vi "Initialize.vi"(7 "timeout, ms (2000)":u32=2000, 8 "error in (no error)":errorcluster, 9 "configuration file path":path, 10 "port":refnum<visa-resource-name>, 11 "SOL MS in":refnum<class "PL SOL Instruments MS.lvclass">) -> (0 "error out":errorcluster, 3 "SOL MS out":refnum<class "PL SOL Instruments MS.lvclass">)   [LabVIEW 2015, in "PL SOL Instruments MS.lvclass"]
doc: "Initializes connection to device using specified settings. <b>Configuration file path</b> is a path to the manufacturer .cfg file (e.g. MS3504.cfg) that contains device specification."
uses:
  PL SOL Instruments MS.lvclass
  PL SOL Instruments MS.lvclass/PL SOL Instruments MS.ctl
  <vilib>/Utility/config.llb/Read Key (U32).vi
  <vilib>/Utility/config.llb/Read Key (String).vi
  <vilib>/Utility/config.llb/Read Key (I32).vi
  <vilib>/Utility/config.llb/NI_LVConfig.lvlib
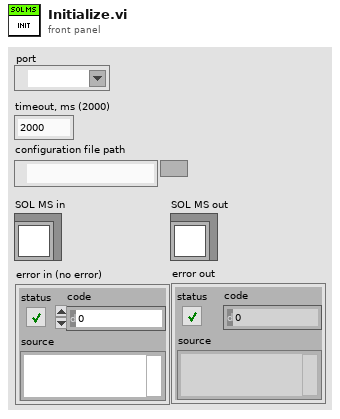
[diagram p1: front panel]
types:
  T1 = typedef "NI_LVConfig.lvlib/Config Data RefNum.ctl" = refnum<k1>
  T2 = cluster{"name":string, "step timeout, ms":u32, "reset timeout, ms":u32, "gratings":cluster{"name":string, "step timeout, ms":u32, "reset timeout, ms":u32, "turret position":i32, "reset position":i32, "max position":i32, "backlash distance":i32, "step size, rad":dbl, "groove density, g/mm":dbl, "theta2, rad":dbl, "blaze wavelength, nm":dbl, "focal length, cm":dbl, "manual change":bool, "manual change position":i32}[], "current grating":cluster{"index":u8, "position":i32}}[]
  T3 = cluster{"name":string, "step timeout, ms":u32, "reset timeout, ms":u32, "gratings":cluster{"name":string, "step timeout, ms":u32, "reset timeout, ms":u32, "turret position":i32, "reset position":i32, "max position":i32, "backlash distance":i32, "step size, rad":dbl, "groove density, g/mm":dbl, "theta2, rad":dbl, "blaze wavelength, nm":dbl, "focal length, cm":dbl, "manual change":bool, "manual change position":i32}[], "current grating":cluster{"index":u8, "position":i32}}
  T4 = cluster{"name":string, "step timeout, ms":u32, "reset timeout, ms":u32, "turret position":i32, "reset position":i32, "max position":i32, "backlash distance":i32, "step size, rad":dbl, "groove density, g/mm":dbl, "theta2, rad":dbl, "blaze wavelength, nm":dbl, "focal length, cm":dbl, "manual change":bool, "manual change position":i32}[]
  T5 = cluster{"name":string, "step timeout, ms":u32, "reset timeout, ms":u32, "turret position":i32, "reset position":i32, "max position":i32, "backlash distance":i32, "step size, rad":dbl, "groove density, g/mm":dbl, "theta2, rad":dbl, "blaze wavelength, nm":dbl, "focal length, cm":dbl, "manual change":bool, "manual change position":i32}
  T6 = cluster{"name":string, "step timeout, ms":u32, "reset timeout, ms":u32, "positions":cluster{"name":string, "position":i32}[], "current position index":u8}[]
  T7 = cluster{"name":string, "step timeout, ms":u32, "reset timeout, ms":u32, "positions":cluster{"name":string, "position":i32}[], "current position index":u8}
  T8 = cluster{"name":string, "step timeout, ms":u32, "reset position":i32, "max position":i32, "backlash distance":i32, "step size, um":dbl, "current position":i32}[]
  T9 = cluster{"name":string, "step timeout, ms":u32, "reset position":i32, "max position":i32, "backlash distance":i32, "step size, um":dbl, "current position":i32}
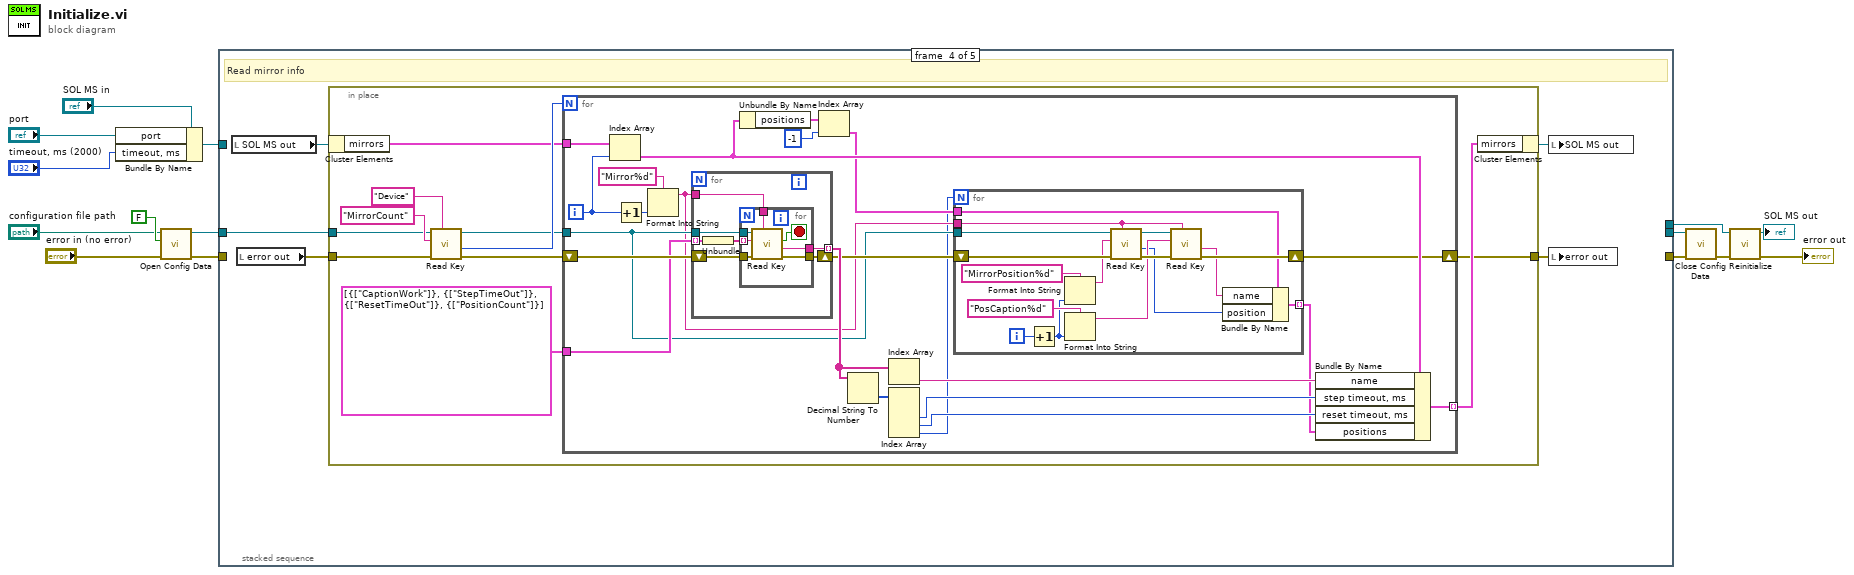
[diagram p0: block diagram]
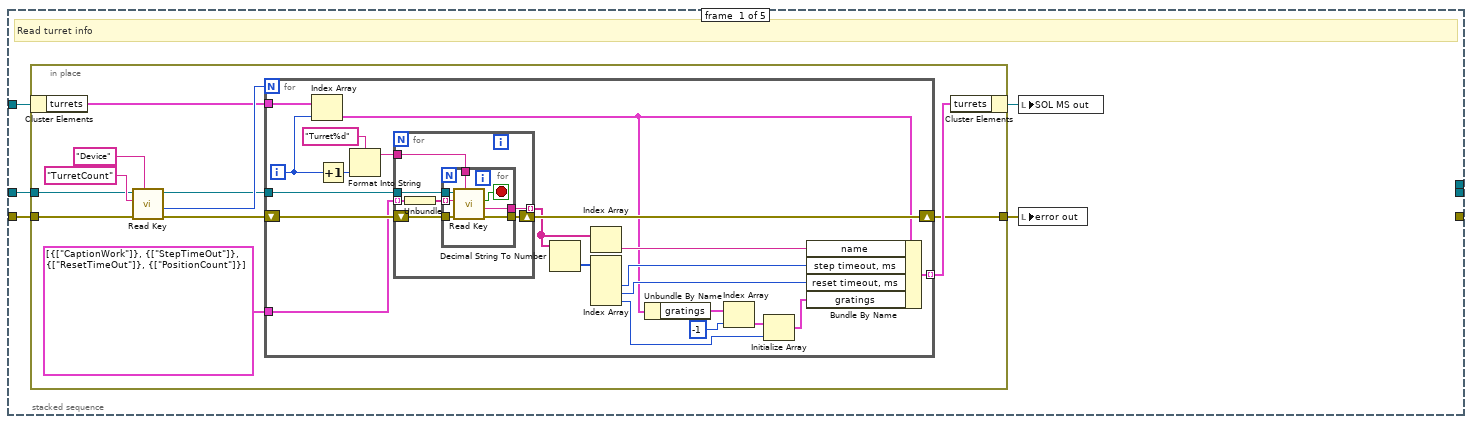
[diagram p2: hidden frame]
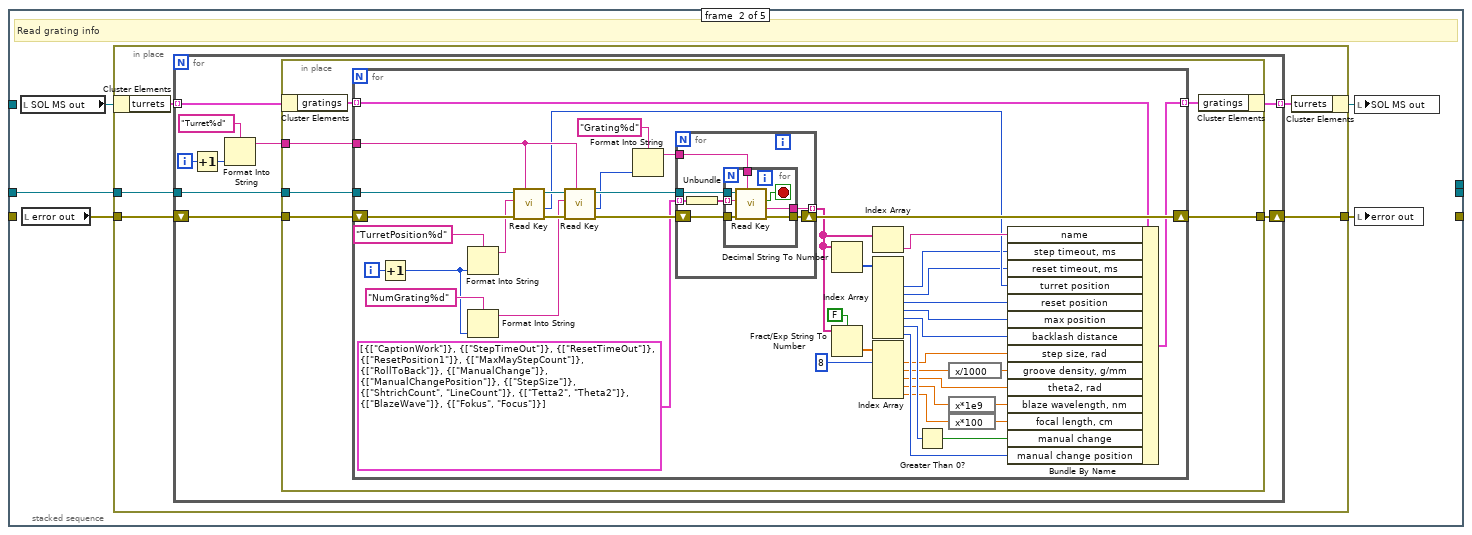
[diagram p3: hidden frame]
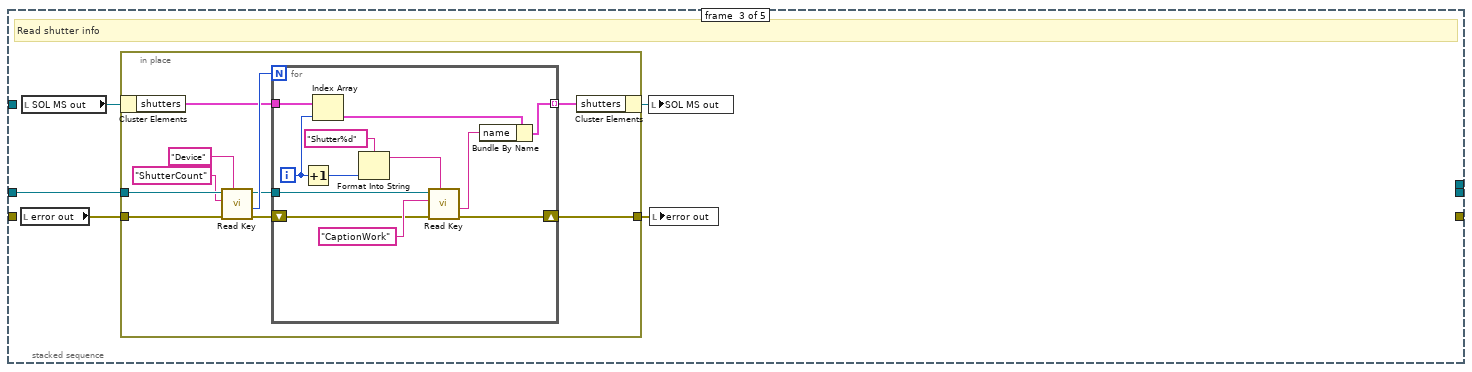
[diagram p4: hidden frame]
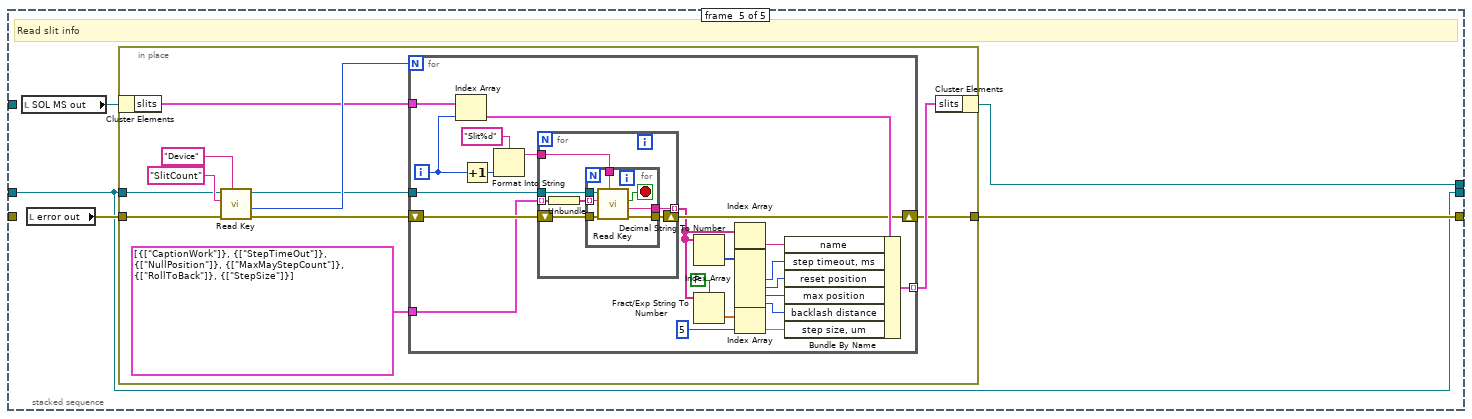
[diagram p5: hidden frame]
diagram:
  n1 = Bundle By Name(cluster="SOL MS in", "port"="port", "timeout, ms"="timeout, ms (2000)") -> (w9:refnum<class "PL SOL Instruments MS.lvclass">)
  n2 = call <vilib>:"Open Config Data.vi"("error in (no error)"="error in (no error)", "create file if necessary (T)"=FALSE, "configuration file path"="configuration file path") -> ("error out"=w8:errorcluster, "refnum"=w2:T1)  [unwired: 6 in, 1 out]
  n3 = stacked-sequence {
    tunnel: w9 -> [w18 _ _ _ _]
    tunnel: w8 -> [w19 _ _ _ _]
    tunnel: [_ _ _ _ w245] -> w5
    tunnel: [_ _ _ _ w246] -> w7
    tunnel: w2 -> [w20 w71 w153 w180 w244]
    tunnel: [_ _ _ _ w244] -> w1
    frame #0 {
      # "Read turret info"
      n4 = in-place {
        in-place-border: w20 -> [w29]
        in-place-border: w19 -> [w28]
        in-place-border: [w21] -> w16
        n5 = in-place-cluster #1(w18) -> ("turrets"=w23:T2)
        n6 = call-poly <vilib>:"Read Key.vi"("section"="Device", "error in (no error)"=w28, "key"="TurretCount", "refnum"=w29) -> ("error out"=w26:errorcluster, "value"=w27:u32, "refnum out"=w25:T1)  [unwired: 4 in, 1 out]
        n7 = for {
          N: w27 -> [_]
          shift-right: [w45] -> w21
          shift-left: w26 -> [w46]
          tunnel: w25 -> [w47]
          tunnel: cluster{string[]}[] [{["CaptionWork"]}, {["StepTimeOut"]}, {["ResetTimeOut"]}, {["PositionCount"]}] -> [w43]
          tunnel: w23 -> [w49]
          tunnel: [w48] -> w22 mode=indexing
          i -> [w50]
          n8 = Index Array(array=w49, index=w50) -> (element=w36:T3)
          n9 = Increment(x=w50) -> (x+1=w52:i32)
          n10 = Format Into String(format string="Turret%d", w52) -> (resulting string=w44:string)  [unwired: 2 in, 1 out]
          n11 = for {
            tunnel: w47 -> [w57]
            shift-right: [w58] -> w45
            shift-left: w46 -> [w59]
            tunnel: w44 -> [w56]
            tunnel: [w55] -> w41 mode=indexing
            tunnel: w43 -> [w53] mode=indexing
            n12 = Unbundle(w53) -> (w54:string[])
            n13 = for {
              tunnel: [w66] -> w58
              tunnel: [w65] -> w55
              tunnel: w59 -> [w64]
              tunnel: w56 -> [w63]
              tunnel: w54 -> [w62] mode=indexing
              tunnel: w57 -> [w60]
              stop <- w61 stop-if-true
              n14 = call-poly <vilib>:"Read Key.vi"("section"=w63, "error in (no error)"=w64, "key"=w62, "refnum"=w60) -> ("error out"=w66:errorcluster, "value"=w65:string, "found?"=w61:bool)  [unwired: 4 in, 1 out]
            }
          }
          n15 = Decimal String To Number(string=w41) -> (number=w40:i32[])  [unwired: 2 in, 1 out]
          n16 = Index Array(array=w41) -> (element=w42:string)  [unwired: 1 in]
          n17 = Index Array(array=w40) -> (element #2=w39:i32, element #3=w38:i32, element #4=w33:i32)  [unwired: 4 in, 1 out]
          n18 = Unbundle By Name(w36) -> ("gratings"=w37:T4)
          n19 = Index Array(array=w37, index=-1) -> (element=w34:T5)
          n20 = Initialize Array(w34, w33) -> (w32:T4)
          n21 = Bundle By Name(cluster=w36, "name"=w42, "step timeout, ms"=w39, "reset timeout, ms"=w38, "gratings"=w32) -> (w48:T3)
        }
        n22 = in-place-cluster #1("turrets"=w22) -> (w17:refnum<class "PL SOL Instruments MS.lvclass">)
      }
      n23 = local write "SOL MS out"(w17) -> ()
      n24 = local write "error out"(w16) -> ()
    }
    frame #1 {
      # "Read grating info"
      n25 = local read "SOL MS out"() -> (w67:refnum<class "PL SOL Instruments MS.lvclass">)
      n26 = local read "error out"() -> (w68:errorcluster)
      n27 = in-place {
        in-place-border: w71 -> [w74]
        in-place-border: w68 -> [w73]
        in-place-border: [w75] -> w69
        n28 = in-place-cluster #2(w67) -> ("turrets"=w76:T2)
        n29 = for {
          shift-right: [w83] -> w75
          shift-left: w73 -> [w84]
          tunnel: w74 -> [w85]
          tunnel: w76 -> [w82] mode=indexing
          tunnel: [w77] -> w72 mode=indexing
          i -> [w79]
          n30 = Increment(x=w79) -> (x+1=w80:i32)
          n31 = Format Into String(format string="Turret%d", w80) -> (resulting string=w78:string)  [unwired: 2 in, 1 out]
          n32 = in-place {
            in-place-border: w85 -> [w91]
            in-place-border: w84 -> [w90]
            in-place-border: [w89] -> w83
            in-place-border: w78 -> [w87]
            n33 = in-place-cluster #3(w82) -> ("gratings"=w88:T4)
            n34 = for {
              tunnel: w91 -> [w124]
              shift-right: [w133] -> w89
              shift-left: w90 -> [w121]
              tunnel: w88 -> [w126] mode=indexing
              tunnel: w87 -> [w120]
              tunnel: [w125] -> w86 mode=indexing
              i -> [w129]
              n35 = Increment(x=w129) -> (x+1=w127:i32)
              n36 = Format Into String(format string="TurretPosition%d", w127) -> (resulting string=w119:string)  [unwired: 2 in, 1 out]
              n37 = Format Into String(format string="NumGrating%d", w127) -> (resulting string=w118:string)  [unwired: 2 in, 1 out]
              n38 = call-poly <vilib>:"Read Key.vi"("section"=w120, "error in (no error)"=w121, "key"=w119, "refnum"=w124) -> ("error out"=w122:errorcluster, "value"=w110:i32, "refnum out"=w123:T1)  [unwired: 4 in, 1 out]
              n39 = call-poly <vilib>:"Read Key.vi"("section"=w120, "error in (no error)"=w122, "key"=w118, "refnum"=w123) -> ("error out"=w117:errorcluster, "value"=w92:u32, "refnum out"=w116:T1)  [unwired: 4 in, 1 out]
              n40 = Format Into String(format string="Grating%d", w92) -> (resulting string=w132:string)  [unwired: 2 in, 1 out]
              n41 = for {
                tunnel: w116 -> [w139]
                shift-right: [w140] -> w133
                shift-left: w117 -> [w141]
                tunnel: w132 -> [w138]
                tunnel: [w137] -> w112 mode=indexing
                tunnel: cluster{string[]}[] [{["CaptionWork"]}, {["StepTimeOut"]}, {["ResetTimeOut"]}, {["ResetPosition1"]}, {["MaxMayStepCount"]}, {["RollToBack"]}, {["ManualChange"]}, {["ManualChangePosition"]}, {["StepSize"]}, {["ShtrichCount", "LineCount"]}, {["Tetta2", "Theta2"]}, {["BlazeWave"]}, {["Fokus", "Focus"]}] -> [w135] mode=indexing
                n42 = Unbundle(w135) -> (w136:string[])
                n43 = for {
                  tunnel: [w148] -> w140
                  tunnel: [w147] -> w137
                  tunnel: w141 -> [w146]
                  tunnel: w138 -> [w145]
                  tunnel: w136 -> [w144] mode=indexing
                  tunnel: w139 -> [w142]
                  stop <- w143 stop-if-true
                  n44 = call-poly <vilib>:"Read Key.vi"("section"=w145, "error in (no error)"=w146, "key"=w144, "refnum"=w142) -> ("error out"=w148:errorcluster, "value"=w147:string, "found?"=w143:bool)  [unwired: 4 in, 1 out]
                }
              }
              n45 = Decimal String To Number(string=w112) -> (number=w131:i32[])  [unwired: 2 in, 1 out]
              n46 = Fract/Exp String To Number(use system decimal point (T)=FALSE, string=w112) -> (number=w113:dbl[])  [unwired: 2 in, 1 out]
              n47 = Index Array(array=w112) -> (element=w114:string)  [unwired: 1 in]
              n48 = Index Array(array=w131) -> (element #2=w109:i32, element #3=w108:i32, element #4=w107:i32, element #5=w106:i32, element #6=w105:i32, element #7=w103:i32, element #8=w104:i32)  [unwired: 8 in, 1 out]
              n49 = Index Array(array=w113, index #1=8 ("index")) -> (element #1=w100:dbl, element #2=w96:dbl, element #3=w95:dbl, element #4=w94:dbl, element #5=w93:dbl)  [unwired: 4 in]
              n50 = Greater Than 0?(x=w103) -> (x > 0?=w102:bool)
              n51 = expression code="x/1000"(w96) -> (w99:dbl)
              n52 = expression code="x*1e9"(w94) -> (w98:dbl)
              n53 = expression code="x*100"(w93) -> (w97:dbl)
              n54 = Bundle By Name(cluster=w126, "name"=w114, "step timeout, ms"=w109, "reset timeout, ms"=w108, "turret position"=w110, "reset position"=w107, "max position"=w106, "backlash distance"=w105, "step size, rad"=w100, "groove density, g/mm"=w99, "theta2, rad"=w95, "blaze wavelength, nm"=w98, "focal length, cm"=w97, "manual change"=w102, "manual change position"=w104) -> (w125:T5)
            }
            n55 = in-place-cluster #3("gratings"=w86) -> (w77:T3)
          }
        }
        n56 = in-place-cluster #2("turrets"=w72) -> (w70:refnum<class "PL SOL Instruments MS.lvclass">)
      }
      n57 = local write "SOL MS out"(w70) -> ()
      n58 = local write "error out"(w69) -> ()
    }
    frame #2 {
      # "Read shutter info"
      n59 = local read "error out"() -> (w152:errorcluster)
      n60 = local read "SOL MS out"() -> (w150:refnum<class "PL SOL Instruments MS.lvclass">)
      n61 = in-place {
        in-place-border: w153 -> [w163]
        in-place-border: [w158] -> w151
        in-place-border: w152 -> [w157]
        n62 = in-place-cluster #4(w150) -> ("shutters"=w156:cluster{"name":string, "is open":bool}[])
        n63 = call-poly <vilib>:"Read Key.vi"("section"="Device", "error in (no error)"=w157, "key"="ShutterCount", "refnum"=w163) -> ("error out"=w159:errorcluster, "value"=w160:u32, "refnum out"=w154:T1)  [unwired: 4 in, 1 out]
        n64 = for {
          N: w160 -> [_]
          tunnel: w156 -> [w167]
          tunnel: [w172] -> w155 mode=indexing
          shift-right: [w169] -> w158
          shift-left: w159 -> [w171]
          tunnel: w154 -> [w164]
          i -> [w166]
          n65 = Increment(x=w166) -> (x+1=w173:i32)
          n66 = Index Array(array=w167, index=w166) -> (element=w165:cluster{"name":string, "is open":bool})
          n67 = Format Into String(format string="Shutter%d", w173) -> (resulting string=w170:string)  [unwired: 2 in, 1 out]
          n68 = call-poly <vilib>:"Read Key.vi"("section"=w170, "error in (no error)"=w171, "key"="CaptionWork", "refnum"=w164) -> ("error out"=w169:errorcluster, "value"=w168:string)  [unwired: 4 in, 2 out]
          n69 = Bundle By Name(cluster=w165, "name"=w168) -> (w172:cluster{"name":string, "is open":bool})
        }
        n70 = in-place-cluster #4("shutters"=w155) -> (w149:refnum<class "PL SOL Instruments MS.lvclass">)
      }
      n71 = local write "SOL MS out"(w149) -> ()
      n72 = local write "error out"(w151) -> ()
    }
    frame #3 {
      # "Read mirror info"
      n73 = local read "SOL MS out"() -> (w177:refnum<class "PL SOL Instruments MS.lvclass">)
      n74 = local read "error out"() -> (w176:errorcluster)
      n75 = in-place {
        in-place-border: w180 -> [w189]
        in-place-border: w176 -> [w188]
        in-place-border: [w181] -> w178
        n76 = in-place-cluster #5(w177) -> ("mirrors"=w183:T6)
        n77 = call-poly <vilib>:"Read Key.vi"("section"="Device", "error in (no error)"=w188, "key"="MirrorCount", "refnum"=w189) -> ("error out"=w186:errorcluster, "value"=w187:u32, "refnum out"=w185:T1)  [unwired: 4 in, 1 out]
        n78 = for {
          N: w187 -> [_]
          shift-right: [w194] -> w181
          shift-left: w186 -> [w208]
          tunnel: w185 -> [w197]
          tunnel: cluster{string[]}[] [{["CaptionWork"]}, {["StepTimeOut"]}, {["ResetTimeOut"]}, {["PositionCount"]}] -> [w207]
          tunnel: w183 -> [w210]
          tunnel: [w209] -> w182 mode=indexing
          i -> [w211]
          n79 = Index Array(array=w210, index=w211) -> (element=w200:T7)
          n80 = Increment(x=w211) -> (x+1=w213:i32)
          n81 = Format Into String(format string="Mirror%d", w213) -> (resulting string=w196:string)  [unwired: 2 in, 1 out]
          n82 = for {
            tunnel: w197 -> [w234]
            shift-right: [w235] -> w198
            shift-left: w208 -> [w236]
            tunnel: w196 -> [w230]
            tunnel: [w233] -> w205 mode=indexing
            tunnel: w207 -> [w231] mode=indexing
            n83 = Unbundle(w231) -> (w232:string[])
            n84 = for {
              tunnel: [w243] -> w235
              tunnel: [w242] -> w233
              tunnel: w236 -> [w241]
              tunnel: w230 -> [w240]
              tunnel: w232 -> [w239] mode=indexing
              tunnel: w234 -> [w237]
              stop <- w238 stop-if-true
              n85 = call-poly <vilib>:"Read Key.vi"("section"=w240, "error in (no error)"=w241, "key"=w239, "refnum"=w237) -> ("error out"=w243:errorcluster, "value"=w242:string, "found?"=w238:bool)  [unwired: 4 in, 1 out]
            }
          }
          n86 = Unbundle By Name(w200) -> ("positions"=w201:cluster{"name":string, "position":i32}[])
          n87 = Index Array(array=w201, index=-1) -> (element=w195:cluster{"name":string, "position":i32})
          n88 = Decimal String To Number(string=w205) -> (number=w204:i32[])  [unwired: 2 in, 1 out]
          n89 = Index Array(array=w205) -> (element=w206:string)  [unwired: 1 in]
          n90 = Index Array(array=w204) -> (element #2=w203:i32, element #3=w202:i32, element #4=w192:i32)  [unwired: 4 in, 1 out]
          n91 = for {
            N: w192 -> [_]
            shift-right: [w222] -> w194
            shift-left: w198 -> [w224]
            tunnel: w195 -> [w221]
            tunnel: w196 -> [w220]
            tunnel: [w219] -> w193 mode=indexing
            tunnel: w197 -> [w214]
            i -> [w228]
            n92 = Increment(x=w228) -> (x+1=w226:i32)
            n93 = Format Into String(format string="MirrorPosition%d", w226) -> (resulting string=w218:string)  [unwired: 2 in, 1 out]
            n94 = Format Into String(format string="PosCaption%d", w226) -> (resulting string=w217:string)  [unwired: 2 in, 1 out]
            n95 = call-poly <vilib>:"Read Key.vi"("section"=w220, "error in (no error)"=w224, "key"=w218, "refnum"=w214) -> ("error out"=w223:errorcluster, "value"=w215:i32, "refnum out"=w225:T1)  [unwired: 4 in, 1 out]
            n96 = call-poly <vilib>:"Read Key.vi"("section"=w220, "error in (no error)"=w223, "key"=w217, "refnum"=w225) -> ("error out"=w222:errorcluster, "value"=w216:string)  [unwired: 4 in, 2 out]
            n97 = Bundle By Name(cluster=w221, "name"=w216, "position"=w215) -> (w219:cluster{"name":string, "position":i32})
          }
          n98 = Bundle By Name(cluster=w200, "name"=w206, "step timeout, ms"=w203, "reset timeout, ms"=w202, "positions"=w193) -> (w209:T7)
        }
        n99 = in-place-cluster #5("mirrors"=w182) -> (w179:refnum<class "PL SOL Instruments MS.lvclass">)
      }
      n100 = local write "SOL MS out"(w179) -> ()
      n101 = local write "error out"(w178) -> ()
    }
    frame #4 {
      # "Read slit info"
      n102 = local read "SOL MS out"() -> (w248:refnum<class "PL SOL Instruments MS.lvclass">)
      n103 = local read "error out"() -> (w247:errorcluster)
      n104 = in-place {
        in-place-border: w244 -> [w257]
        in-place-border: w247 -> [w256]
        in-place-border: [w249] -> w245
        n105 = in-place-cluster #6(w248) -> ("slits"=w251:T8)
        n106 = call-poly <vilib>:"Read Key.vi"("section"="Device", "error in (no error)"=w256, "key"="SlitCount", "refnum"=w257) -> ("error out"=w254:errorcluster, "value"=w255:u32, "refnum out"=w253:T1)  [unwired: 4 in, 1 out]
        n107 = for {
          N: w255 -> [_]
          shift-right: [w267] -> w249
          shift-left: w254 -> [w276]
          tunnel: w253 -> [w269]
          tunnel: cluster{string[]}[] [{["CaptionWork"]}, {["StepTimeOut"]}, {["NullPosition"]}, {["MaxMayStepCount"]}, {["RollToBack"]}, {["StepSize"]}] -> [w275]
          tunnel: w251 -> [w278]
          tunnel: [w277] -> w250 mode=indexing
          i -> [w279]
          n108 = Index Array(array=w278, index=w279) -> (element=w270:T9)
          n109 = Increment(x=w279) -> (x+1=w281:i32)
          n110 = Format Into String(format string="Slit%d", w281) -> (resulting string=w268:string)  [unwired: 2 in, 1 out]
          n111 = for {
            tunnel: w269 -> [w286]
            shift-right: [w287] -> w267
            shift-left: w276 -> [w288]
            tunnel: w268 -> [w282]
            tunnel: [w285] -> w264 mode=indexing
            tunnel: w275 -> [w283] mode=indexing
            n112 = Unbundle(w283) -> (w284:string[])
            n113 = for {
              tunnel: [w295] -> w287
              tunnel: [w294] -> w285
              tunnel: w288 -> [w293]
              tunnel: w282 -> [w292]
              tunnel: w284 -> [w291] mode=indexing
              tunnel: w286 -> [w289]
              stop <- w290 stop-if-true
              n114 = call-poly <vilib>:"Read Key.vi"("section"=w292, "error in (no error)"=w293, "key"=w291, "refnum"=w289) -> ("error out"=w295:errorcluster, "value"=w294:string, "found?"=w290:bool)  [unwired: 4 in, 1 out]
            }
          }
          n115 = Decimal String To Number(string=w264) -> (number=w273:i32[])  [unwired: 2 in, 1 out]
          n116 = Fract/Exp String To Number(use system decimal point (T)=FALSE, string=w264) -> (number=w265:dbl[])  [unwired: 2 in, 1 out]
          n117 = Index Array(array=w264) -> (element=w274:string)  [unwired: 1 in]
          n118 = Index Array(array=w273) -> (element #2=w272:i32, element #3=w271:i32, element #4=w266:i32, element #5=w260:i32)  [unwired: 5 in, 1 out]
          n119 = Index Array(array=w265, index=5) -> (element=w261:dbl)
          n120 = Bundle By Name(cluster=w270, "name"=w274, "step timeout, ms"=w272, "reset position"=w271, "max position"=w266, "backlash distance"=w260, "step size, um"=w261) -> (w277:T9)
        }
        n121 = in-place-cluster #6("slits"=w250) -> (w246:refnum<class "PL SOL Instruments MS.lvclass">)
      }
    }
  }
  n122 = call <vilib>:"Close Config Data.vi"("error in (no error)"=w5, "refnum"=w1) -> ("error out"=w4:errorcluster)  [unwired: 8 in, 1 out]
  n123 = call "Reinitialize.vi"("error in (no error)"=w4, "SOL MS in"=w7) -> ("error out"=→"error out":errorcluster, "SOL MS out"=→"SOL MS out":refnum<class "PL SOL Instruments MS.lvclass">)  [unwired: 8 in]
